vi "emi_Write Keys.vi"(0 "Ini Path(..app../config.ini)":path=path "", 1 "Section":string, 5 "Key Names":string[](array[string]), 7 "Values":variant[](array[variant]), 11 "error in (no error)":errorcluster) -> (6 "file created?":bool, 15 "error out":errorcluster)   [LabVIEW 2011]
doc: "Write numerous keys into ini file. Creates and openes ini file id \\\\s needed"
uses:
  App/emi_Application Folder.vi
  <vilib>/Utility/libraryn.llb/Check if File or Folder Exists.vi
  <vilib>/Utility/config.llb/NI_LVConfig.lvlib
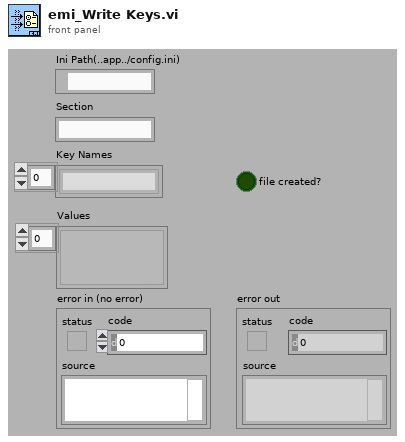
[diagram p1: front panel]
types:
  T1 = typedef "NI_LVConfig.lvlib/Config Data RefNum.ctl" = refnum<k1>
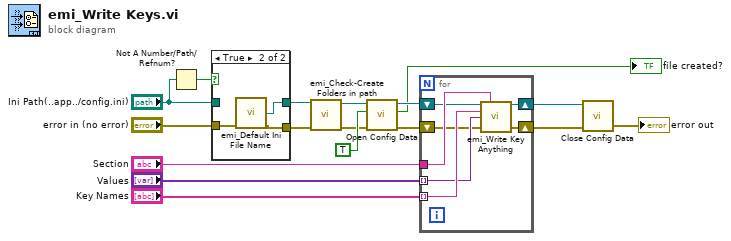
[diagram p0: block diagram]
diagram:
  n1 = Not A Number/Path/Refnum?(number/path/refnum="Ini Path(..app../config.ini)") -> (NaN/Path/Refnum?=w7:bool)
  n2 = case shown="True" w7 {
    tunnel: [w19 w21] -> w4
    tunnel: "Ini Path(..app../config.ini)" -> [w19 _]
    tunnel: "error in (no error)" -> [w18 w22]
    tunnel: [w18 w20] -> w5
    frame False {
    }
    frame True {
      n3 = call "emi_Default Ini File Name.vi"("error in (no error)"=w22) -> ("Path"=w21:path, "error out"=w20:errorcluster)  [unwired: 13 in]
    }
  }
  n4 = call "emi_Check-Create Folders in path.vi"("Path including file"=w4, "error in (no error)"=w5) -> ("Path out"=w2:path, "error out"=w3:errorcluster)  [unwired: 11 in, 1 out]
  n5 = call <vilib>:"Open Config Data.vi"("error in (no error)"=w3, "create file if necessary (T)"=TRUE, "configuration file path"=w2) -> ("error out"=w12:errorcluster, "file created?"=→"file created?":bool, "refnum"=w13:T1)  [unwired: 6 in]
  n6 = for {
    tunnel: "Section" -> [w29]
    tunnel: "Values" -> [w26] mode=indexing
    tunnel: "Key Names" -> [w27] mode=indexing
    shift-right: [w24] -> w10
    shift-left: w12 -> [w25]
    shift-right: [w23] -> w11
    shift-left: w13 -> [w28]
    n7 = call "emi_Write Key Anything.vi"("Ini file refnum"=w28, "Section(Default)"=w29, "Name"=w27, "Anything"=w26, "error in (no error)"=w25) -> ("Ini file refnum out"=w23:T1, "error out"=w24:errorcluster)  [unwired: 9 in]
  }
  n8 = call <vilib>:"Close Config Data.vi"("error in (no error)"=w10, "refnum"=w11) -> ("error out"=→"error out":errorcluster)  [unwired: 8 in, 1 out]
